vi "Fake Theory.vi"(11 "Condition":bool) -> (0 "error out":errorcluster)   [LabVIEW 2017, in "LVUnit Test Executor.Tests.lvlib"]
uses:
  LVUnit Test Executor.Tests.lvlib
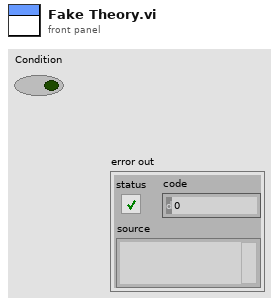
[diagram p1: front panel]
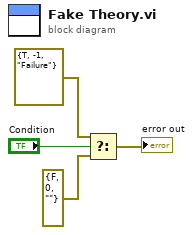
[diagram p0: block diagram]
diagram:
  n1 = Select(t=errorcluster {"status"=TRUE, "code"=-1, "source"="Failure"} ("error constant"), s="Condition", f=errorcluster {"status"=FALSE, "code"=0, "source"=""}) -> (s? t:f=→"error out":errorcluster)
